vi "scan_Bias.vi"() -> ()   [LabVIEW 2011, in "run.lvlib"]
doc: "I. Description:\nThis example demonstrates how to continuously output a waveform using an internal sample clock and a digital start trigger.\n\nII. Instructions for Running:\n1. Select the Physical Channel to correspond to where your signal is output on the DAQ device.\n2. Enter the Minimum and Maximum Voltage Ranges.\n3. Specify the Desired Frequency of the output Waveform\n4. Select the Digital Trigger Source.\n5. Specify the desired Trigger Edge.\n6. Enter the Waveform Information. See the documentation of the Waveform Buffer Generation SubVI for information on each parameter.\n\nIII. Block Diagram Steps:\n1. Create an Analog Output Voltage Task\n2.Call the DAQmx Timing (Use Waveform) VI which sets the sample clock rate based on the input waveform parameters, and set the sample mode to Continuous.\n3. Define the Triggering parameters: Source and Edge\n4. Write the waveform to the output buffer.\n5. Call the Start VI.\n6. Loop continuously until the user presses the Stop button. Check for errors every 100 ms using the Is Task Done? VI\n7. Call the Clear Task VI to clear the Task.\n8. Use the popup dialog box to display an error or warning if any.\n\nIV. I/O Connections Overview:\nMake sure your signal output terminal matches the Physical Channel I/O Control. Also, make sure your digital trigger terminal matches the Trigger Source Control. For further connection information, refer to your hardware reference manual."
uses:
  Hal/testing/run.lvlib
  <vilib>/Utility/error.llb/DialogType.ctl
  <vilib>/DAQmx/write.llb/DAQmx Write (Analog 1D Wfm NChan NSamp).vi
  <vilib>/DAQmx/create/channels.llb/DAQmx Create Channel (AO-Voltage-Basic).vi
  <vilib>/DAQmx/configure/timing.llb/DAQmx Timing (Use Waveform).vi
  <vilib>/DAQmx/miscellaneous.llb/DAQmx Fill In Error Info.vi
panel:
  in  "Uwire":bool=TRUE
  in  "Bias":bool=TRUE
  in  "updown":bool=TRUE
  in  "Amplitude U":dbl=2.5 caption="Amplitude Current U" format="%0.2p"
  in  "offset U":dbl=22.5
  in  "Amplitude bias":dbl=0.2 caption="Amplitude Current Bias" format="%0.2p"
  in  "offset Bias":dbl=2.0
  in  "offset Updown (Amp)":dbl=2.6
  out "Resulting Frequency":dbl format="%.2f"
  in  "Cycles per Buffer":i32=15
  in  "Waveform Type":T1(ring)
  in  "Amplitude UpDown":dbl=0.2 caption="Amplitude Current Updown" format="%0.2p"
  in  "Samples per Buffer":dbl=750.0
  in  "Desired Frequency":dbl=0.1 format="%.2f"
  out "Output Waveform":waveform(dbl)[](graph) caption="Output bias"
  in  "Physical Channels":tag="Ao8b/ao2:4"
  in  "Minimum Value":dbl=-10.0 format="%0.2f"
  in  "Maximum Value":dbl=10.0 format="%0.2f"
  in  "stop":bool
  # "For instructions, select Help>>Show Context Help"
  # "Channel Parameters"
  # "Timing Parameters"
  # "Waveform Information"
  # "Updown : Ao2"
  # "Bias : Ao3"
  # "UWire : Ao4"
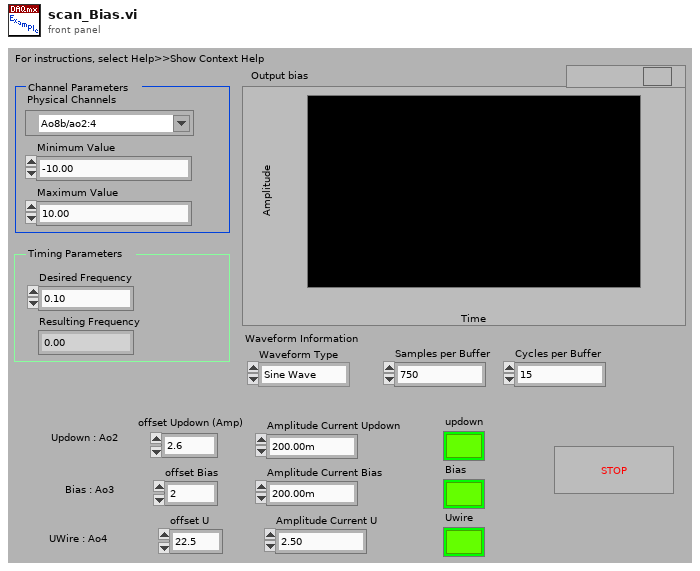
[diagram p1: front panel]
types:
  T1 = enum16{"Sine Wave", "Triangle Wave", "Square Wave", "Sawtooth Wave"}
  T2 = typedef "DialogType.ctl" = u16
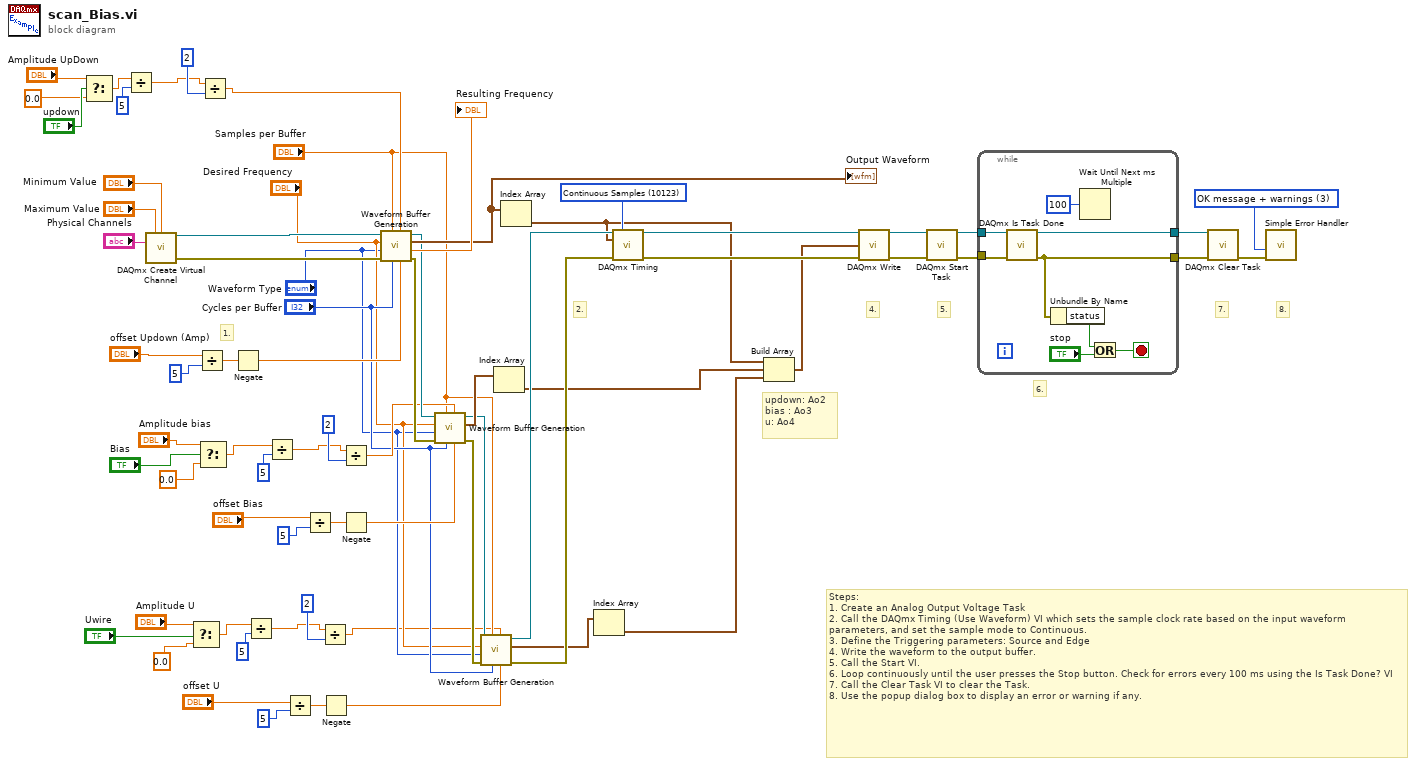
[diagram p0: block diagram]
diagram:
  w62 = T2 3 items=["no dialog", "OK message", "continue or stop message", "OK message + warnings", "continue/stop + warnings"] ("type of dialog (OK msg:1)")
  w69 = 10123 items=["Finite Samples"=10178, "Continuous Samples"=10123] ("sample mode")
  # "updown: Ao2\nbias : Ao3\nu: Ao4"
  # "8."
  # "6."
  # "7."
  # "Steps: \n1. Create an Analog Output Voltage Task\n2. Call the DAQmx Timing (Use Waveform) VI which sets the sample clock rate based on the input waveform parameters, and set the sample mode to Continuous.\n3. Define the Triggering parameters: Source and Edge\n4. Write the waveform to the output buffer.\n5. Call the Start VI.\n6. Loop continuously until the user presses the Stop button. Check for errors every 100 ms using the Is Task Done? VI\n7. Call the Clear Task VI to clear the Task.\n8. Use the popup dialog box to display an error or warning if any."
  # "5."
  # "4."
  # "2."
  # "1."
  n1 = Select(t="Amplitude UpDown", s="updown", f=0.0) -> (s? t:f=w7:dbl)
  n2 = Divide(x=w7, y=5) -> (x/y=w48:dbl)
  n3 = call-poly <vilib>:"DAQmx Create Virtual Channel.vi"("maximum value"="Maximum Value", "minimum value"="Minimum Value", "physical channels"="Physical Channels") -> ("task out"=w46:refnum<k21>, "error out"=w58:errorcluster)  [unwired: 11 in]
  n4 = Select(t="Amplitude U", s="Uwire", f=0.0) -> (s? t:f=w3:dbl)
  n5 = Divide(x="offset Updown (Amp)", y=5) -> (x/y=w51:dbl)
  n6 = Select(t="Amplitude bias", s="Bias", f=0.0) -> (s? t:f=w10:dbl)
  n7 = Divide(x=w48, y=2) -> (x/y=w49:dbl)
  n8 = Negate(x=w51) -> (-x=w50:dbl)
  n9 = Divide(x=w3, y=5) -> (x/y=w33:dbl)
  n10 = Divide(x=w10, y=5) -> (x/y=w44:dbl)
  n11 = Divide(x="offset U", y=5) -> (x/y=w30:dbl)
  n12 = Divide(x="offset Bias", y=5) -> (x/y=w41:dbl)
  n13 = Divide(x=w33, y=2) -> (x/y=w18:dbl)
  n14 = Negate(x=w30) -> (-x=w22:dbl)
  n15 = Divide(x=w44, y=2) -> (x/y=w24:dbl)
  n16 = Negate(x=w41) -> (-x=w38:dbl)
  n17 = call "Waveform Buffer Generation.vi"("offset"=w50, "Amplitude"=w49, "Cycles per Buffer"="Cycles per Buffer", "Samples per Buffer"="Samples per Buffer", "error in (no error)"=w58, "Waveform Type"="Waveform Type", "Desired Frequency"="Desired Frequency", "task/channels in"=w46) -> ("error out"=w37:errorcluster, "Resulting Frequency"=→"Resulting Frequency":dbl, "Waveform"=w56:waveform(dbl)[], "task out"=w39:refnum<k21>)
  "Output Waveform" <- w56
  n18 = call "Waveform Buffer Generation.vi"("offset"=w38, "Amplitude"=w24, "Cycles per Buffer"="Cycles per Buffer", "Samples per Buffer"="Samples per Buffer", "error in (no error)"=w37, "Waveform Type"="Waveform Type", "Desired Frequency"="Desired Frequency", "task/channels in"=w39) -> ("error out"=w26:errorcluster, "Waveform"=w36:waveform(dbl)[], "task out"=w28:refnum<k21>)  [unwired: 1 out]
  n19 = call "Waveform Buffer Generation.vi"("offset"=w22, "Amplitude"=w18, "Cycles per Buffer"="Cycles per Buffer", "Samples per Buffer"="Samples per Buffer", "error in (no error)"=w26, "Waveform Type"="Waveform Type", "Desired Frequency"="Desired Frequency", "task/channels in"=w28) -> ("error out"=w25:errorcluster, "Waveform"=w17:waveform(dbl)[], "task out"=w27:refnum<k21>)  [unwired: 1 out]
  n20 = Index Array(array=w36) -> (element=w14:waveform(dbl))  [unwired: 1 in]
  n21 = Index Array(array=w56) -> (element=w15:waveform(dbl))  [unwired: 1 in]
  n22 = Index Array(array=w17) -> (element=w16:waveform(dbl))  [unwired: 1 in]
  n23 = call-poly <vilib>:"DAQmx Timing.vi"("task/channels in"=w27, "sample mode"=w69, "waveform"=w15, "error in"=w25) -> ("task out"=w55:refnum<k21>, "error out"=w54:errorcluster)  [unwired: 10 in]
  n24 = Build Array(w15, w14, w16) -> (w35:waveform(dbl)[])
  n25 = call-poly <vilib>:"DAQmx Write.vi"("task/channels in"=w55, "data"=w35, "error in"=w54) -> ("task out"=w66:refnum<k21>, "error out"=w65:errorcluster)  [unwired: 10 in, 1 out]
  n26 = call <vilib>:"DAQmx Start Task.vi"("task/channels in"=w66, "error in"=w65) -> ("task out"=w70:refnum<k21>, "error out"=w64:errorcluster)  [unwired: 12 in]
  n27 = while {
    tunnel: w70 -> [w74]
    tunnel: [w71] -> w60
    tunnel: w64 -> [w73]
    tunnel: [w72] -> w59
    stop <- w78 stop-if-true
    n28 = call <vilib>:"DAQmx Is Task Done.vi"("task/channels in"=w74, "error in"=w73) -> ("task out"=w71:refnum<k21>, "error out"=w72:errorcluster)  [unwired: 11 in, 1 out]
    n29 = Unbundle By Name(w72) -> ("status"=w76:bool)
    n30 = Wait Until Next ms Multiple(millisecond multiple=u32 100) -> ()  [unwired: 1 out]
    n31 = Or(x=w76, y="stop") -> (x .or. y?=w78:bool)
  }
  n32 = call <vilib>:"DAQmx Clear Task.vi"("task in"=w60, "error in"=w59) -> ("error out"=w61:errorcluster)  [unwired: 13 in]
  n33 = call <vilib>:"Simple Error Handler.vi"("type of dialog (OK msg:1)"=w62, "error in (no error)"=w61) -> ()  [unwired: 3 in, 5 out]
